vi "Pose3DTranslate.vi"(9 "Translation Vector":T1, 11 "Starting Pose":T2) -> (3 "Resulting Pose":T2)   [LabVIEW 2018]
uses:
  Pose3D.ctl
  Vector/Vector3D.ctl
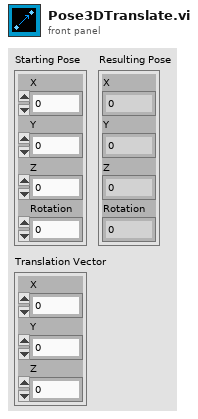
[diagram p1: front panel]
types:
  T1 = typedef "Vector3D.ctl" = cluster{"X":dbl, "Y":dbl, "Z":dbl}
  T2 = typedef "Pose3D.ctl" = cluster{"X":dbl, "Y":dbl, "Z":dbl, "Rotation":dbl}
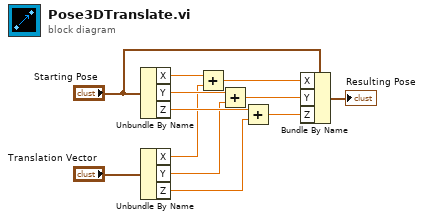
[diagram p0: block diagram]
diagram:
  n1 = Unbundle By Name("Starting Pose") -> ("X"=w11:dbl, "Y"=w7:dbl, "Z"=w6:dbl)
  n2 = Unbundle By Name("Translation Vector") -> ("X"=w3:dbl, "Y"=w2:dbl, "Z"=w1:dbl)
  n3 = Add(x=w11, y=w3) -> (x+y=w8:dbl)
  n4 = Add(x=w7, y=w2) -> (x+y=w4:dbl)
  n5 = Add(x=w6, y=w1) -> (x+y=w5:dbl)
  n6 = Bundle By Name(cluster="Starting Pose", "X"=w8, "Y"=w4, "Z"=w5) -> (→"Resulting Pose":T2)
